vi "fgv_Gslam_config.vi"(7 "cmd":T3, 11 "G config":T2) -> (3 "G cofnig out":T2)   [LabVIEW 2019]
uses:
  Ctrl/cmd_common.ctl
  <vilib>/Analysis/Matrix/Datatypes/RealMatrix.ctl
  <vilib>/Analysis/Matrix/NI_Matrix.lvlib
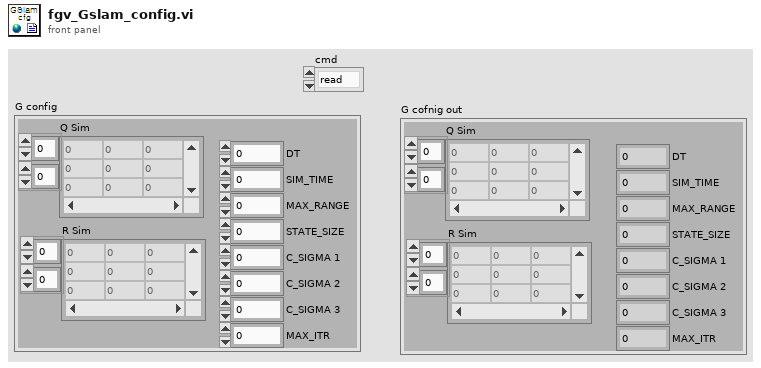
[diagram p1: front panel]
types:
  T1 = typedef "NI_Matrix.lvlib/RealMatrix.ctl" = dbl[][]
  T2 = cluster{"Q Sim":T1, "R Sim":T1, "DT":dbl, "SIM_TIME":dbl, "MAX_RANGE":dbl, "STATE_SIZE":i32, "C_SIGMA 1":dbl, "C_SIGMA 2":dbl, "C_SIGMA 3":dbl, "MAX_ITR":u32}
  T3 = typedef "cmd_common.ctl" = enum16{"read", "write"}
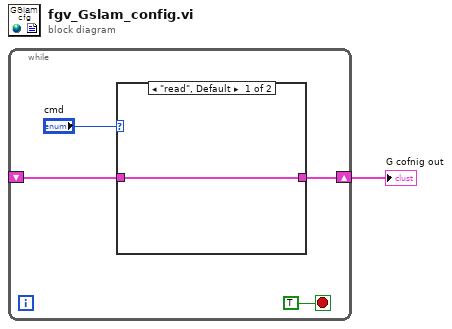
[diagram p0: block diagram]
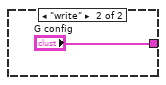
[diagram p2: hidden frame]
diagram:
  n1 = while {
    shift-right: [w3] -> w1
    shift-left: _ -> [w2]
    stop <- TRUE stop-if-true
    n2 = case shown="\"read\", Default" "cmd" {
      tunnel: [w6 "G config"] -> w3
      tunnel: w2 -> [w6 _]
      frame "read", Default {
      }
      frame "write" {
      }
    }
  }
  "G cofnig out" <- w1
